vi "Power Peak Bounds Detector.vi"(2 "df":dbl, 3 "Signal In":waveform(dbl)) -> (0 "min":dbl, 1 "max":dbl)   [LabVIEW 2013]
uses:
  <vilib>/measure/mamon.llb/Waveform Peak Detection for 1 Chan.vi
  <vilib>/measure/NI_MAPro.lvlib
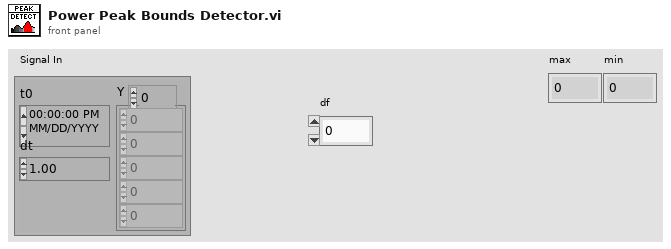
[diagram p1: front panel]
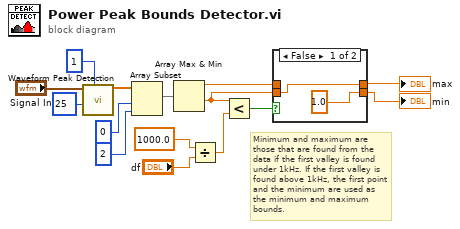
[diagram p0: block diagram]
diagram:
  # "Minimum and maximum are those that are found from the data if the first valley is found under 1kHz. If the first valley is found above 1kHz, the first point and the minimum are used as the minimum and maximum bounds."
  n1 = call-poly <vilib>:"Waveform Peak Detection.vi"("peaks/valleys"=1, "width"=25, "Signal In"="Signal In") -> ("Locations"=w14:dbl[])  [unwired: 4 in, 4 out]
  n2 = Array Subset(array=w14, index=0, length=2) -> (w10:dbl[])
  n3 = Array Max & Min(array=w10) -> (max value=w3:dbl, min value=w4:dbl)  [unwired: 2 out]
  n4 = Divide(x=1000.0, y="df") -> (x/y=w6:dbl)
  n5 = Less?(x=w4, y=w6) -> (x < y?=w5:bool)
  n6 = case shown="False" w5 {
    tunnel: w4 -> [w17 w18]
    tunnel: w3 -> [_ w19]
    tunnel: [w17 w19] -> w2
    tunnel: [1.0 ("Numeric") w18] -> w1
    frame False {
    }
    frame True {
    }
  }
  "max" <- w2
  "min" <- w1
